vi "InterpolateWristPositions.vi"(1 "MiddlePoints":T2[](array[typedef]), 2 "SubsequentPose":T1, 3 "PriorPose":T1) -> (0 "ConvertedPoints":T1[](array[typedef]))   [LabVIEW 2018]
uses:
  TypeDefs/ArmAbsolutePosition.ctl
  ArgosLib/Path Planning/TypeDefs/Point2D.ctl
  ArgosLib/ArgosLib.lvlib
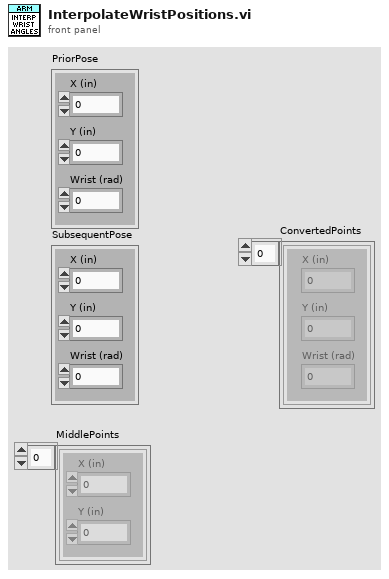
[diagram p1: front panel]
types:
  T1 = typedef "ArmAbsolutePosition.ctl" = cluster{"X (in)":dbl, "Y (in)":dbl, "Wrist (rad)":dbl}
  T2 = typedef "ArgosLib.lvlib/Point2D.ctl" = cluster{"X (in)":dbl, "Y (in)":dbl}
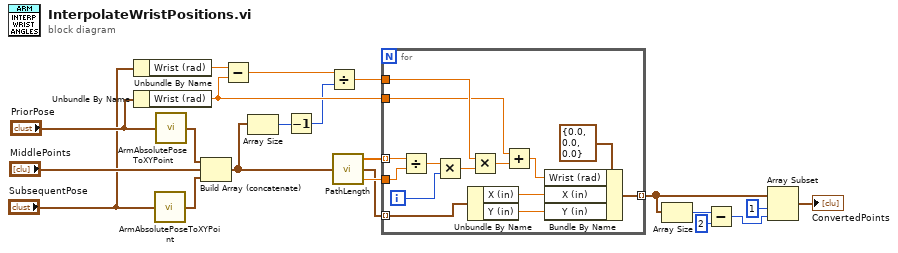
[diagram p0: block diagram]
diagram:
  n1 = Unbundle By Name("SubsequentPose") -> ("Wrist (rad)"=w14:dbl)
  n2 = Unbundle By Name("PriorPose") -> ("Wrist (rad)"=w13:dbl)
  n3 = call "ArmAbsolutePoseToXYPoint.vi"("ArmAbsolutePose"="SubsequentPose") -> ("2DPoint"=w19:T2)
  n4 = call "ArmAbsolutePoseToXYPoint.vi"("ArmAbsolutePose"="PriorPose") -> ("2DPoint"=w21:T2)
  n5 = Build Array (concatenate)(w21, "MiddlePoints", w19) -> (w11:T2[])
  n6 = Subtract(x=w14, y=w13) -> (x-y=w12:dbl)
  n7 = Array Size(array=w11) -> (size(s)=w10:i32)
  n8 = Decrement(x=w10) -> (x-1=w9:i32)
  n9 = Divide(x=w12, y=w9) -> (x/y=w8:dbl)
  n10 = call "PathLength.vi"("PathIn"=w11) -> ("Path Length"=w15:dbl, "PathOut"=w7:T2[], "IndexedPathLength"=w16:dbl[])  [unwired: 2 in]
  n11 = for {
    tunnel: w16 -> [w35] mode=indexing
    tunnel: w13 -> [w28]
    tunnel: w15 -> [w34]
    tunnel: w8 -> [w30]
    tunnel: w7 -> [w27] mode=indexing
    tunnel: [w22] -> w5 mode=indexing
    i -> [w32]
    n12 = Divide(x=w35, y=w34) -> (x/y=w33:dbl)
    n13 = Multiply(x=w33, y=w32) -> (x*y=w31:dbl)
    n14 = Unbundle By Name(w27) -> ("X (in)"=w24:dbl, "Y (in)"=w23:dbl)
    n15 = Multiply(x=w30, y=w31) -> (x*y=w29:dbl)
    n16 = Add(x=w28, y=w29) -> (x+y=w25:dbl)
    n17 = Bundle By Name(cluster=T1 {"X (in)"=0.0, "Y (in)"=0.0, "Wrist (rad)"=0.0} ("PriorPose"), "Wrist (rad)"=w25, "X (in)"=w24, "Y (in)"=w23) -> (w22:T1)
  }
  n18 = Array Size(array=w5) -> (size(s)=w3:i32)
  n19 = Subtract(x=w3, y=2) -> (x-y=w1:i32)
  n20 = Array Subset(array=w5, index=1, length=w1) -> (→"ConvertedPoints":T1[])
